vi "FUG_PowerSupply.set device state.vi"(0 "i ref in":refnum<vi>, 1 "deviceState":T1 items=["ERROR"=-1, "OK"=0, "NOT_OK"=1], 2 "implicit":bool, 3 "ms timeout (10000)":i32=10000, 4 "device error":errorcluster, 5 "error in (no error)":errorcluster, 7 "mayResetError (FALSE)":bool) -> (14 "i ref out":refnum<vi>, 17 "timed out":bool, 19 "error out":errorcluster)   [LabVIEW 2014, in "FUG_PowerSupply.lvlib"]
doc: "This is an override method to take care of class specific stuff in the \"calculation\" of the device state.\n\nSets the state of a device. There are three device states\n\n0 : OK\n>0: NOT_OK\n<0: ERROR \n\nIn case the device state is set \"implicitely\", the severity of the \"device error\" is analyzed. In case of \"fatal\" or \"error\", the device state is set to \"ERROR\". In case of \"warning\", the device state is set to \"NOT_OK\". In all other cases, the device state is set to \"OK\".\n\nPer default, the device state can not be changed in case of \"ERROR\". If one wants to reset the device state one has to call THIS method with the option mayResetError set to TRUE."
uses:
  FUG_PowerSupply.lvlib
  CSCore/CSApplicationBaseClasses/DeviceBase/DeviceBase.deviceState.ctl
  CSCore/CSApplicationBaseClasses/PSChannelBase/PSChannelBase.statusType.ctl
  CSCore/CSApplicationBaseClasses/PSChannelBase/PSChannelBase.serviceType.ctl
  CSCore/CSApplicationBaseClasses/PSChannelBase/PSChannelBase.directionType.ctl
  CSCore/CSApplicationBaseClasses/DeviceBase/DeviceBase.lvlib
  CSCore/CSApplicationBaseClasses/PSChannelBase/PSChannelBase.lvlib
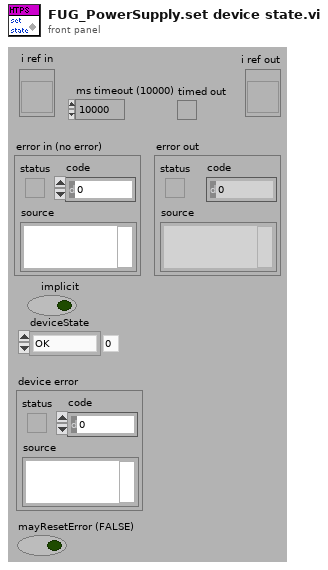
[diagram p1: front panel]
types:
  T1 = typedef "DeviceBase.lvlib/DeviceBase.deviceState.ctl" = i16
  T2 = typedef "PSChannelBase.lvlib/PSChannelBase.directionType.ctl" = enum16{"unknown", "update actual value", "update nominal value", "update both"}
  T3 = typedef "PSChannelBase.lvlib/PSChannelBase.serviceType.ctl" = enum16{"onOff", "voltage", "current", "tripCurrent", "rampUpSpeed", "rampDownSpeed", "status"}
  T4 = typedef "PSChannelBase.lvlib/PSChannelBase.statusType.ctl" = i32
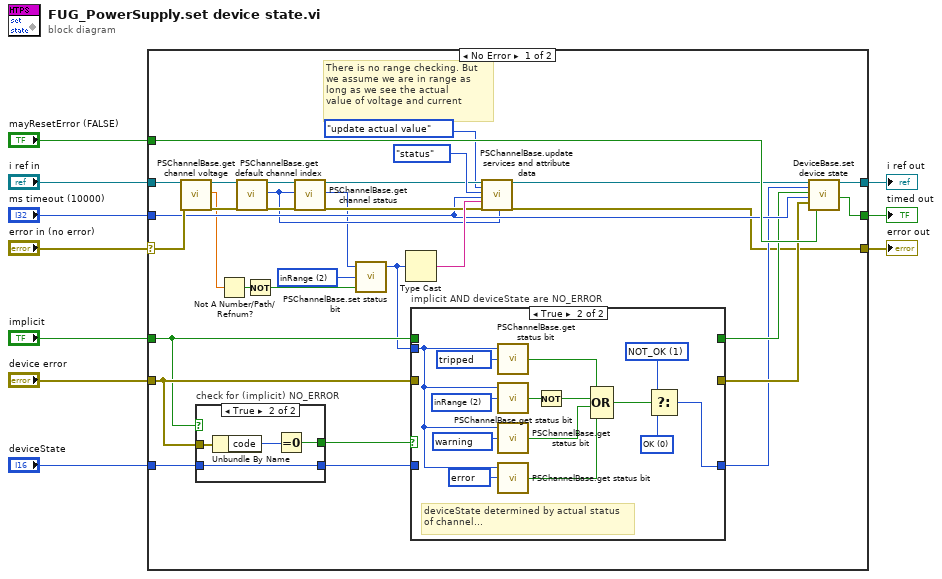
[diagram p0: block diagram]
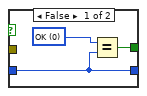
[diagram p3: hidden frame]
diagram:
  n1 = case shown="No Error" "error in (no error)" {
    selector: "error in (no error)" -> [w39 w67]
    tunnel: [w41 _] -> w10
    tunnel: [w15 w68] -> w9
    tunnel: "ms timeout (10000)" -> [w32 _]
    tunnel: "implicit" -> [w21 _]
    tunnel: "i ref in" -> [w40 w68]
    tunnel: "device error" -> [w24 _]
    tunnel: "deviceState" -> [w26 _]
    tunnel: [w16 w67] -> w2
    tunnel: "mayResetError (FALSE)" -> [w42 _]
    frame No Error {
      w34 = T4 2 items=["onOff"=1, "inRange"=2, "rampingUp"=4, "rampingDown"=8, "currentRegulated"=16, "voltageRegulated"=32, "reserved1"=64, "reserved2"=128, "reserved3"=256, "reserved4"=512, "reserved5"=1024, "reserved6"=2048, "reserved7"=4096, "reserved8"=8192, "reserved9"=16384, "reserved10"=32768, "reserved11"=65536, "user1"=131072, "user2"=262144, "user3"=524288, "user4"=1048576, "user5"=2097152, "user6"=4194304, "user7"=8388608, "user8"=16777216, "user9"=33554432, "user10"=67108864, "user11"=134217728, "tripped"=268435456, "warning"=536870912, "error"=1073741824] ("statusBit")
      # "There is no range checking. But\nwe assume we are in range as\nlong as we see the actual\nvalue of voltage and current"
      n2 = call "PSChannelBase.get channel voltage.vi"("i ref in"=w40, "error in (no error)"=w39) -> ("i ref out"=w31:refnum<vi>, "voltage"=w13:dbl, "error out"=w29:errorcluster)  [unwired: 15 in]
      n3 = case "check for (implicit) NO_ERROR" shown="True" w21 {
        tunnel: w24 -> [_ w66]
        tunnel: [w61 w64] -> w25
        tunnel: w26 -> [w60 w63]
        tunnel: [w60 w63] -> w23
        frame False {
          w62 = T1 0 items=["ERROR"=-1, "OK"=0, "NOT_OK"=1] ("x")
          n4 = Equal?(x=w62, y=w60) -> (x = y?=w61:bool)
        }
        frame True {
          n5 = Unbundle By Name(w66) -> ("code"=w65:i32)
          n6 = Equal To 0?(x=w65) -> (x = 0?=w64:bool)
        }
      }
      n7 = Not A Number/Path/Refnum?(number/path/refnum=w13) -> (NaN/Path/Refnum?=w12:bool)
      n8 = call "PSChannelBase.get default channel index.vi"("i ref in"=w31, "error in (no error)"=w29) -> ("i ref out"=w30:refnum<vi>, "defaultChannelIndex"=w27:i32, "error out"=w28:errorcluster)  [unwired: 15 in]
      n9 = Not(x=w12) -> (.not. x?=w11:bool)
      n10 = call "PSChannelBase.get channel status.vi"("i ref in"=w30, "channelIndex"=w27, "error in (no error)"=w28) -> ("i ref out"=w35:refnum<vi>, "status"=w18:i32, "error out"=w37:errorcluster)  [unwired: 14 in]
      n11 = call "PSChannelBase.set status bit.vi"("set"=w11, "statusBit"=w34, "status"=w18) -> ("status out"=w14:T4)  [unwired: 2 in]
      n12 = Type Cast(x=w14) -> (*(type *) &x=w38:string)  [unwired: 1 in]
      n13 = case "implicit AND deviceState are NO_ERROR" shown="True" w25 {
        tunnel: w24 -> [w44 _]
        tunnel: w23 -> [w45 _]
        tunnel: [w45 w46] -> w19
        tunnel: [w44 _] -> w22
        tunnel: w21 -> [w43 _]
        tunnel: [w43 _] -> w20
        tunnel: w14 -> [_ w56]
        frame False {
        }
        frame True {
          w47 = T1 1 items=["ERROR"=-1, "OK"=0, "NOT_OK"=1] ("t")
          w48 = T1 0 items=["ERROR"=-1, "OK"=0, "NOT_OK"=1] ("deviceState")
          w55 = T4 1073741824 items=["onOff"=1, "inRange"=2, "rampingUp"=4, "rampingDown"=8, "currentRegulated"=16, "voltageRegulated"=32, "reserved1"=64, "reserved2"=128, "reserved3"=256, "reserved4"=512, "reserved5"=1024, "reserved6"=2048, "reserved7"=4096, "reserved8"=8192, "reserved9"=16384, "reserved10"=32768, "reserved11"=65536, "user1"=131072, "user2"=262144, "user3"=524288, "user4"=1048576, "user5"=2097152, "user6"=4194304, "user7"=8388608, "user8"=16777216, "user9"=33554432, "user10"=67108864, "user11"=134217728, "tripped"=268435456, "warning"=536870912, "error"=1073741824] ("statusBit")
          w57 = T4 536870912 items=["onOff"=1, "inRange"=2, "rampingUp"=4, "rampingDown"=8, "currentRegulated"=16, "voltageRegulated"=32, "reserved1"=64, "reserved2"=128, "reserved3"=256, "reserved4"=512, "reserved5"=1024, "reserved6"=2048, "reserved7"=4096, "reserved8"=8192, "reserved9"=16384, "reserved10"=32768, "reserved11"=65536, "user1"=131072, "user2"=262144, "user3"=524288, "user4"=1048576, "user5"=2097152, "user6"=4194304, "user7"=8388608, "user8"=16777216, "user9"=33554432, "user10"=67108864, "user11"=134217728, "tripped"=268435456, "warning"=536870912, "error"=1073741824] ("statusBit")
          w58 = T4 2 items=["onOff"=1, "inRange"=2, "rampingUp"=4, "rampingDown"=8, "currentRegulated"=16, "voltageRegulated"=32, "reserved1"=64, "reserved2"=128, "reserved3"=256, "reserved4"=512, "reserved5"=1024, "reserved6"=2048, "reserved7"=4096, "reserved8"=8192, "reserved9"=16384, "reserved10"=32768, "reserved11"=65536, "user1"=131072, "user2"=262144, "user3"=524288, "user4"=1048576, "user5"=2097152, "user6"=4194304, "user7"=8388608, "user8"=16777216, "user9"=33554432, "user10"=67108864, "user11"=134217728, "tripped"=268435456, "warning"=536870912, "error"=1073741824] ("statusBit")
          w59 = T4 268435456 items=["onOff"=1, "inRange"=2, "rampingUp"=4, "rampingDown"=8, "currentRegulated"=16, "voltageRegulated"=32, "reserved1"=64, "reserved2"=128, "reserved3"=256, "reserved4"=512, "reserved5"=1024, "reserved6"=2048, "reserved7"=4096, "reserved8"=8192, "reserved9"=16384, "reserved10"=32768, "reserved11"=65536, "user1"=131072, "user2"=262144, "user3"=524288, "user4"=1048576, "user5"=2097152, "user6"=4194304, "user7"=8388608, "user8"=16777216, "user9"=33554432, "user10"=67108864, "user11"=134217728, "tripped"=268435456, "warning"=536870912, "error"=1073741824] ("statusBit")
          # "deviceState determined by actual status\nof channel..."
          n14 = call "PSChannelBase.get status bit.vi"("statusBit"=w59, "status"=w56) -> ("set"=w54:bool)  [unwired: 3 in]
          n15 = call "PSChannelBase.get status bit.vi"("statusBit"=w58, "status"=w56) -> ("set"=w51:bool)  [unwired: 3 in]
          n16 = call "PSChannelBase.get status bit.vi"("statusBit"=w57, "status"=w56) -> ("set"=w52:bool)  [unwired: 3 in]
          n17 = call "PSChannelBase.get status bit.vi"("statusBit"=w55, "status"=w56) -> ("set"=w53:bool)  [unwired: 3 in]
          n18 = Not(x=w51) -> (.not. x?=w50:bool)
          n19 = Compound Arithmetic op=OR(w54, w50, w52, w53) -> (w49:bool)
          n20 = Select(t=w47, s=w49, f=w48) -> (s? t:f=w46:T1)
        }
      }
      n21 = call "PSChannelBase.update services and attribute data.vi"("i ref in"=w35, "direction"=PSChannelBase.directionType."update actual value", "service"=PSChannelBase.serviceType."status", "ms timeout (10000)"=w32, "value"=w38, "error in (no error)"=w37, "channelNumber"=w27) -> ("i ref out"=w17:refnum<vi>, "error out"=w16:errorcluster)  [unwired: 10 in, 1 out]
      n22 = call "DeviceBase.set device state.vi"("i ref in"=w17, "deviceState"=w19, "implicit"=w20, "ms timeout (10000)"=w32, "device error"=w22, "mayResetError (FALSE)"=w42) -> ("i ref out"=w15:refnum<vi>, "timed out"=w41:bool)  [unwired: 11 in, 1 out]
    }
    frame Error {
    }
  }
  "error out" <- w2
  "i ref out" <- w9
  "timed out" <- w10
